vi "Attach Global Fixture.vi"(8 "error in (no error)":errorcluster, 10 "Global Fixture Test Case":refnum<class "Global Fixture Test Case.lvclass">) -> (0 "error out":errorcluster, 3 "Global Fixture Test Suite Out":refnum<class "Global Fixture Test Suite.lvclass">)   [LabVIEW 2020, in "Global Fixture Test Suite.lvclass"]
uses:
  Global Fixture Test Suite.lvclass
  Global Fixture Test Case/Global Fixture Test Case.lvclass
  Global Fixture Test Suite.lvclass/Global Fixture Test Suite.ctl
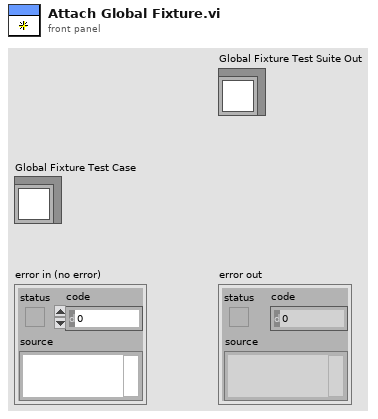
[diagram p1: front panel]
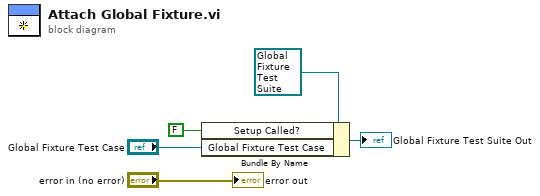
[diagram p0: block diagram]
diagram:
  n1 = Bundle By Name(cluster=refnum<class "Global Fixture Test Suite.lvclass"> refnum ("Test Suite with Global Fixture"), "Setup Called?"=FALSE, "Global Fixture Test Case"="Global Fixture Test Case") -> (→"Global Fixture Test Suite Out":refnum<class "Global Fixture Test Suite.lvclass">)
  "error out" <- "error in (no error)"
